vi "OOK_FrameBuild.vi"(11 "input bit stream":i8[](array[numeric])) -> (3 "output bit stream":i8[](array[numeric]))   [LabVIEW 2014]
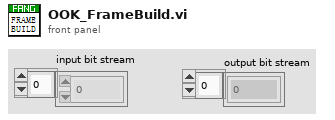
[diagram p1: front panel]
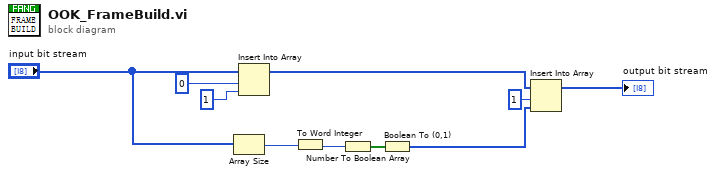
[diagram p0: block diagram]
diagram:
  n1 = Array Size(array="input bit stream") -> (size(s)=w7:i32)
  n2 = Insert Into Array(array="input bit stream", index=0, new element=i8 1 ("new element/subarray")) -> (w4:i8[])
  n3 = To Word Integer(number=w7) -> (16bit integer=w5:i16)
  n4 = Number To Boolean Array(number=w5) -> (Boolean array=w6:bool[])
  n5 = Boolean To (0,1)(Boolean=w6) -> (0, 1=w3:i16[])
  n6 = Insert Into Array(array=w4, index=1, new element=w3) -> (→"output bit stream":i8[])
